vi "ActionVIOnCompile.vi"(8 "error in (no error)":errorcluster, 11 "Device Item Ref in":T1 format="%.0x") -> (0 "error out":errorcluster)   [LabVIEW 2019, in "Reset Hardware System Explorer.lvlib"]
uses:
  Reset Hardware System Explorer.lvlib
  <vilib>/NI VeriStand/Custom Device Tools/Custom Device Utility Library/Custom Device Utility Library.lvlib
  <vilib>/NI VeriStand/Custom Device Tools/Custom Device Utility Library/NI VeriStand - Search for Item by Name.vi
  <vilib>/NI VeriStand/Custom Device API/Custom Device API.lvlib
  <vilib>/NI VeriStand/Custom Device API/Custom Device Item Ref.ctl
  <vilib>/NI/NIVS Inline Async API/_Data Access System Explorer/Data Access System Explorer.lvlib
  <vilib>/NI VeriStand/Custom Device API/Set Item Property (Variant).vi
  Shared/Compiled.Settings.ctl
  Shared/Reset Hardware Shared.lvlib
  Shared/Constants.vi
  <vilib>/NI/NI VeriStand Advanced SysDef API/SysDef API/Advanced System Definition.lvlib
  <vilib>/NI/NI VeriStand Advanced SysDef API/_SubVIs/SysDef.Property.Get.Boolean.vi
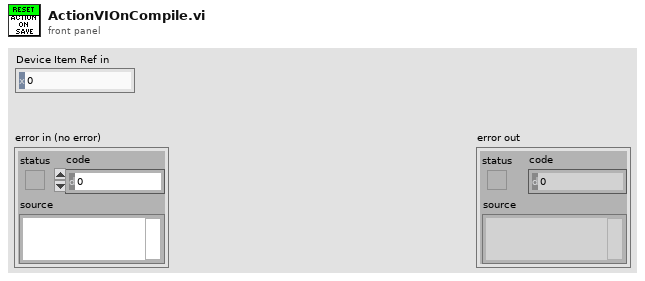
[diagram p1: front panel]
types:
  T1 = typedef "Custom Device API.lvlib/Custom Device Item Ref.ctl" = u64
  T2 = cluster{"Name":string, "Type":enum16{"Output/Write", "Input/Read", "Input/ReadWrite"}, "VS Refs":T1[]}
  T3 = enum16{"Output/Write", "Input/Read", "Input/ReadWrite"}
  T4 = typedef "Reset Hardware Shared.lvlib/Compiled.Settings.ctl" = cluster{"Name":string, "Reset DAQmx AO":bool, "Reset XNET":bool}
  T5 = typedef "Custom Device API.lvlib/Custom Device Item Info.ctl" = cluster{"Name":string, "Is Channel":bool, "GUID":string, "Is Waveform":bool}
  T6 = cluster{"Name":string, "Type":enum16{"Output/Write", "Input/Read", "Input/ReadWrite"}, "VS Refs":T1[]}[]
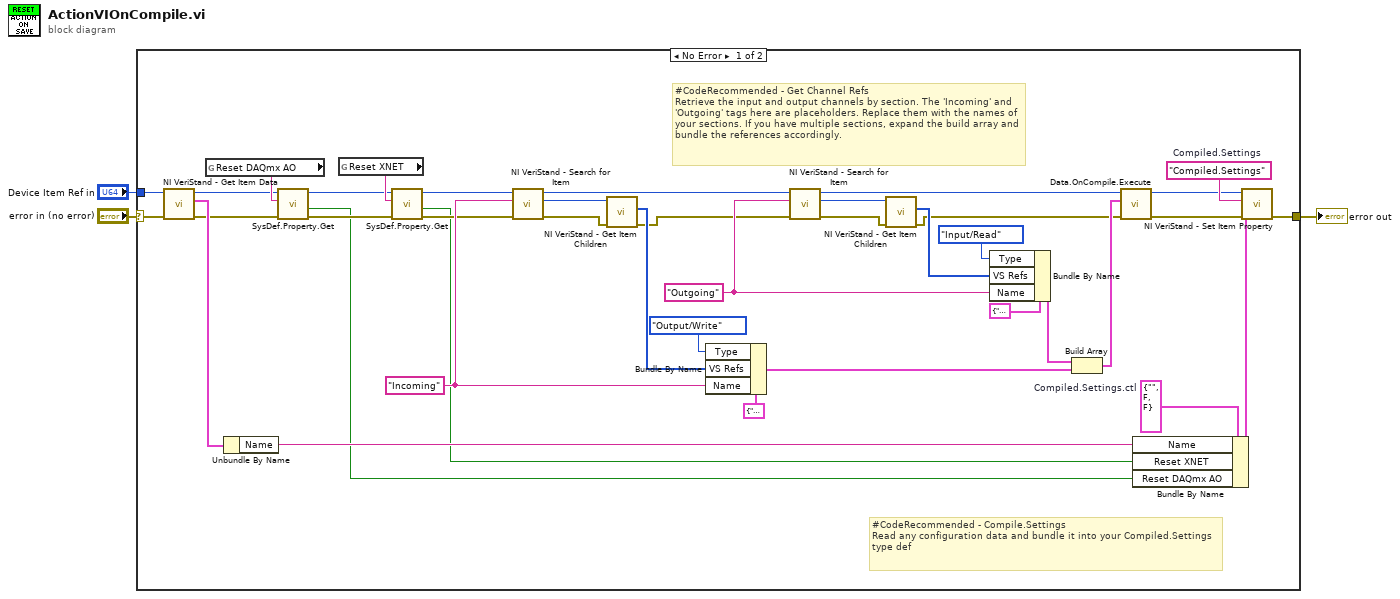
[diagram p0: block diagram]
diagram:
  n1 = case shown="No Error" "error in (no error)" {
    selector: "error in (no error)" -> [w35 w43]
    tunnel: [w36 w43] -> w2
    tunnel: "Device Item Ref in" -> [w34 _]
    frame No Error {
      w14 = T4 {"Name"="", "Reset DAQmx AO"=FALSE, "Reset XNET"=FALSE}  # Compiled.Settings.ctl
      w29 = "Outgoing" ("Item Name")
      w31 = "Incoming" ("Item Name")
      w38 = "Compiled.Settings"  # Compiled.Settings
      # "#CodeRecommended - Get Channel Refs\nRetrieve the input and output channels by section. The 'Incoming' and 'Outgoing' tags here are placeholders. Replace them with the names of your sections. If you have multiple sections, expand the build array and bundle the references accordingly."
      # "#CodeRecommended - Compile.Settings\nRead any configuration data and bundle it into your Compiled.Settings type def"
      n2 = call <vilib>:"NI VeriStand - Get Item Data.vi"("error in (no error)"=w35, "Item Ref in"=w34) -> ("error out"=w7:errorcluster, "Item Info"=w33:T5, "Item Ref out"=w9:T1)  [unwired: 6 in, 1 out]
      n3 = global read "Constants.vi" "Reset DAQmx AO"() -> (w13:string)
      n4 = Unbundle By Name(w33) -> ("Name"=w32:string)
      n5 = call-poly <vilib>:"SysDef.Property.Get.vi"("error in (no error)"=w7, "Property Name"=w13, "nodeID"=w9) -> ("error out"=w10:errorcluster, "Value out"=w5:bool, "nodeID out"=w11:u64)  [unwired: 5 in, 1 out]
      n6 = global read "Constants.vi" "Reset XNET"() -> (w12:string)
      n7 = call-poly <vilib>:"SysDef.Property.Get.vi"("error in (no error)"=w10, "Property Name"=w12, "nodeID"=w11) -> ("error out"=w6:errorcluster, "Value out"=w4:bool, "nodeID out"=w8:u64)  [unwired: 5 in, 1 out]
      n8 = call-poly <vilib>:"NI VeriStand - Search for Item.vi"("error in"=w6, "Item Name"=w31, "Section Ref in"=w8) -> ("error out"=w42:errorcluster, "Item Ref"=w41:T1, "Section Ref out"=w18:T1)  [unwired: 5 in, 1 out]
      n9 = call <vilib>:"NI VeriStand - Get Item Children.vi"("error in (no error)"=w42, "Item Ref in"=w41) -> ("error out"=w17:errorcluster, "Child Refs"=w30:T1[])  [unwired: 6 in, 2 out]
      n10 = Bundle By Name(cluster=T2 {"Name"="", "Type"=enum."Output/Write", "VS Refs"=[]} ("Group"), "Type"=T3."Output/Write", "VS Refs"=w30, "Name"=w31) -> (w21:T2)
      n11 = call-poly <vilib>:"NI VeriStand - Search for Item.vi"("error in"=w17, "Item Name"=w29, "Section Ref in"=w18) -> ("error out"=w39:errorcluster, "Item Ref"=w40:T1, "Section Ref out"=w19:T1)  [unwired: 5 in, 1 out]
      n12 = call <vilib>:"NI VeriStand - Get Item Children.vi"("error in (no error)"=w39, "Item Ref in"=w40) -> ("error out"=w20:errorcluster, "Child Refs"=w25:T1[])  [unwired: 6 in, 2 out]
      n13 = Bundle By Name(cluster=T2 {"Name"="", "Type"=enum."Output/Write", "VS Refs"=[]} ("Group"), "Type"=T3."Input/Read", "VS Refs"=w25, "Name"=w29) -> (w27:T2)
      n14 = Build Array(w27, w21) -> (w24:T6)
      n15 = call <vilib>:"Data.OnCompile.Execute.vi"("error in"=w20, "VS Ref Groups"=w24, "Custom Device Ref"=w19) -> ("error out"=w16:errorcluster, "Custom Device Ref"=w15:T1)  [unwired: 7 in]
      n16 = Bundle By Name(cluster=w14, "Name"=w32, "Reset XNET"=w4, "Reset DAQmx AO"=w5) -> (w37:T4)
      n17 = call-poly <vilib>:"NI VeriStand - Set Item Property.vi"("error in (no error)"=w16, "Value"=w37, "Property Name"=w38, "Item Ref in"=w15) -> ("error out"=w36:errorcluster)  [unwired: 5 in, 2 out]
    }
    frame Error {
    }
  }
  "error out" <- w2
